vi "Begin.vi"(8 "error in (no error)":errorcluster, 11 "Comp Driver in":refnum<class "Comp Driver.lvclass">) -> (0 "error out":errorcluster, 3 "Comp Driver out":refnum<class "Comp Driver.lvclass">)   [LabVIEW 2014, in "Comp Driver.lvlib" / "Comp Driver.lvclass"]
uses:
  Comp Driver.lvclass
  Comp Driver.lvclass/Comp Driver.ctl
  Robot/Driver/Driver Class/Driver.lvclass
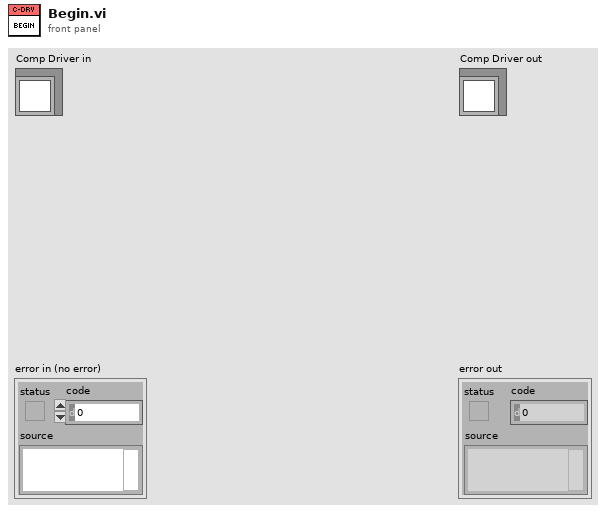
[diagram p1: front panel]
types:
  T1 = typedef "WPI_JoystickDeviceEnum.ctl" = enum16{"USB 0", "USB 1", "USB 2", "USB 3", "USB 4", "USB 5"}
  T2 = typedef "WPI_JoystickDevRef.ctl" = cluster{"Device":T1}
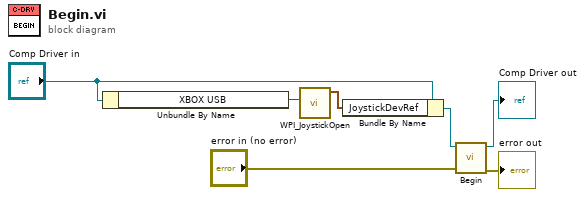
[diagram p0: block diagram]
diagram:
  n1 = Unbundle By Name("Comp Driver in") -> ("XBOX USB"=w5:T1)
  n2 = call <vilib>:"WPI_JoystickOpen.vi"("JoystickDevice"=w5) -> ("JoystickDevRef"=w4:T2)  [unwired: 10 in]
  n3 = Bundle By Name(cluster="Comp Driver in", "JoystickDevRef"=w4) -> (w2:refnum<class "Comp Driver.lvclass">)
  n4 = call-parent "Begin.vi"("error in (no error)"="error in (no error)", "System Actor in"=w2) -> ("error out"=→"error out":errorcluster, "System Actor out"=→"Comp Driver out":refnum<class "Comp Driver.lvclass">)  [unwired: 8 in]
